vi "EnqueueDependency.vi"(8 "error in (no error)":errorcluster, 9 "ILabVIEWItem to enqueue":refnum<class "ILabVIEWItem.lvclass">, 11 "CDependencyQueue in":refnum<class "CDependencyQueue.lvclass">) -> (0 "error out":errorcluster, 3 "CDependencyQueue out":refnum<class "CDependencyQueue.lvclass">)   [LabVIEW 2020, in "DependencyInspection.lvlib" / "CDependencyQueue.lvclass"]
uses:
  CDependencyQueue.lvclass
  obj/Addons/LabVIEWObjectInterfaces.lvlibp/LabVIEWObjectInterfaces/ILabVIEWItem/ILabVIEWItem.lvclass
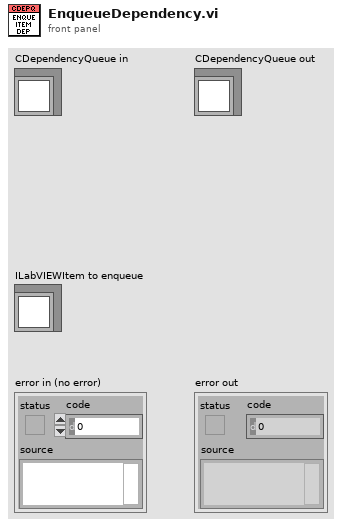
[diagram p1: front panel]
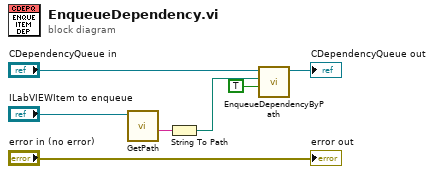
[diagram p0: block diagram]
diagram:
  n1 = call-dynamic "GetPath.vi"("ILabVIEWItem in"="ILabVIEWItem to enqueue") -> ("Path"=w3:string)  [unwired: 8 in, 2 out]
  n2 = String To Path(string=w3) -> (path=w4:path)
  n3 = call-dynamic "EnqueueDependencyByPath.vi"("Shallow deps?"=TRUE, "Path"=w4, "CDependencyQueue in"="CDependencyQueue in") -> ("CDependencyQueue out"=→"CDependencyQueue out":refnum<class "CDependencyQueue.lvclass">)  [unwired: 7 in, 1 out]
  "error out" <- "error in (no error)"
